vi "7Zip.vi"(6 "error in":errorcluster, 7 "Zip file Dir":path caption="Папка, в которую надо сложить архив", 8 "7za Dir":path caption="Папка, в которо лежит 7za.exe архиватор", 9 "File":path caption="Полный путь до файла, который надо зажать") -> (0 "error out":errorcluster, 1 "return code":i32, 2 "standard error":string, 3 "standard output":string="\r\n", 4 "new path":path caption="Полный путь до перемещённого архива файла")   [LabVIEW 2010]
panel:
  # "Инструмент для сжатия файлов архиватором 7za.exe  \nhttp://www.7-zip.org/download.html (нужен для командной строки)\n------------------------------------------------------------------------------------------------\nУказанный файл сжимается архиватором, лежащим по указанному месту\nи переносится в указанную папку. \n\nЕсли файла нет - ошибка\nЕсли архиватора нет - ошибка\nЕсли папки, куда переместить файл нет - ошибка\n\nЕсли всё ок, то в конце нет ошибок и в \"new path: путь до перемещенного \nзажатого файла, который можно дальше отсылать.\n-----------------------------------------------------------------------------------------------\n\nверсия 1.0 \nБутымов Антон Ноябрь 2010"
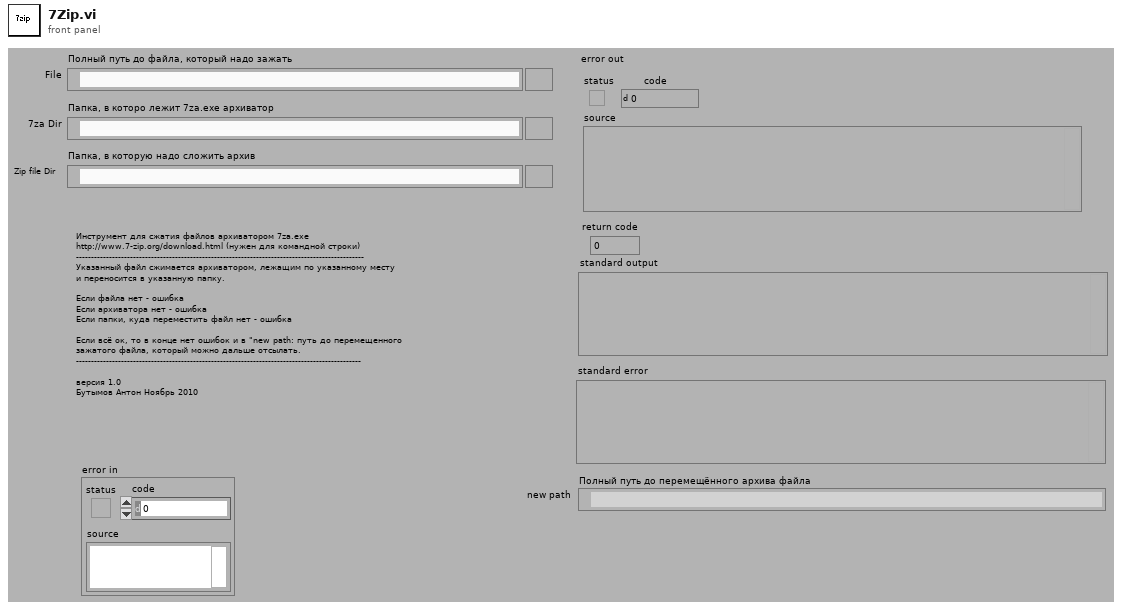
[diagram p1: front panel]
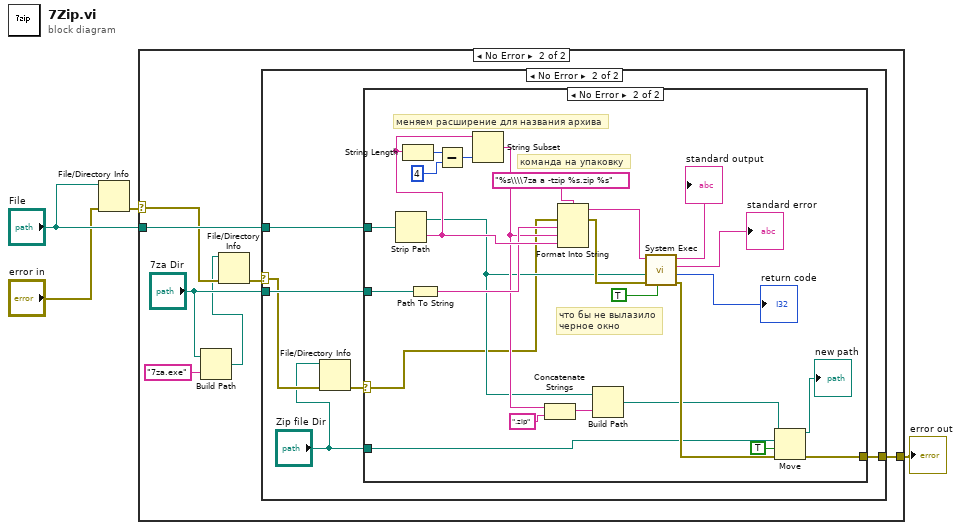
[diagram p0: block diagram]
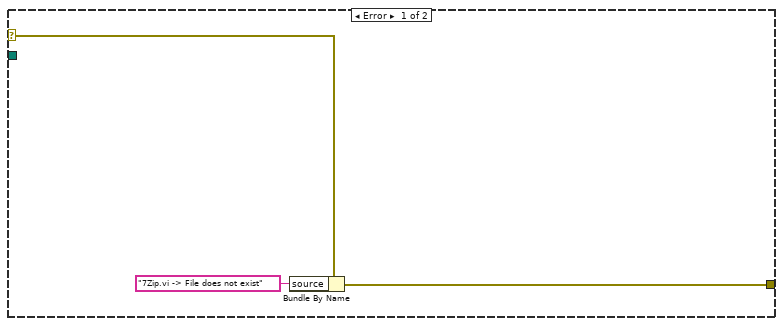
[diagram p2: hidden frame]
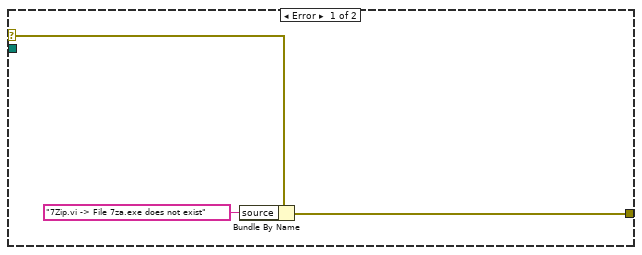
[diagram p3: hidden frame]
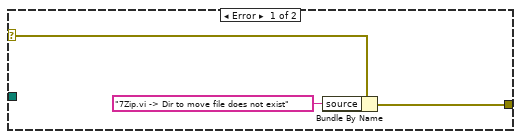
[diagram p4: hidden frame]
diagram:
  n1 = File/Directory Info(path="File", error in="error in") -> (error out=w2:errorcluster)  [unwired: 6 out]
  n2 = case shown="No Error" w2 {
    selector: w2 -> [w6 w12]
    tunnel: [w5 w14] -> w4
    tunnel: "File" -> [_ w13]
    frame Error {
      n3 = Bundle By Name(cluster=w6, "source"="7Zip.vi -> File does not exist") -> (w5:errorcluster)
    }
    frame No Error {
      n4 = Build Path(base path="7za Dir", name or relative path="7za.exe") -> (appended path=w8:path)
      n5 = File/Directory Info(path=w8, error in=w12) -> (error out=w11:errorcluster)  [unwired: 6 out]
      n6 = case shown="No Error" w11 {
        selector: w11 -> [w16 w20]
        tunnel: [w15 w23] -> w14
        tunnel: w13 -> [_ w22]
        tunnel: "7za Dir" -> [_ w21]
        frame Error {
          n7 = Bundle By Name(cluster=w16, "source"="7Zip.vi -> File 7za.exe does not exist") -> (w15:errorcluster)
        }
        frame No Error {
          n8 = File/Directory Info(path="Zip file Dir", error in=w20) -> (error out=w18:errorcluster)  [unwired: 6 out]
          n9 = case shown="No Error" w18 {
            selector: w18 -> [w26 w28]
            tunnel: [w25 w38] -> w23
            tunnel: w22 -> [_ w31]
            tunnel: w21 -> [_ w30]
            tunnel: "Zip file Dir" -> [_ w29]
            frame Error {
              n10 = Bundle By Name(cluster=w26, "source"="7Zip.vi -> Dir to move file does not exist") -> (w25:errorcluster)
            }
            frame No Error {
              # "что бы не вылазило\nчерное окно"
              # "команда на упаковку"
              # "меняем расширение для названия архива"
              n11 = Strip Path(path=w31) -> (stripped path=w34:path, name=w41:string)
              n12 = String Length(string=w41) -> (length=w44:i32)
              n13 = Path To String(path=w30) -> (string=w40:string)
              n14 = Subtract(x=w44, y=4) -> (x-y=w42:i32)
              n15 = String Subset(string=w41, length (rest)=w42) -> (substring=w37:string)  [unwired: 1 in]
              n16 = Concatenate Strings(w37, ".zip" ("string")) -> (w35:string)
              n17 = Format Into String(format string="%s\\\\7za a -tzip %s.zip %s" ("command line"), error in=w28, w40, w37, w41) -> (resulting string=w45:string, error out=w46:errorcluster)  [unwired: 1 in]
              n18 = Build Path(base path=w34, name or relative path=w35) -> (appended path=w33:path)
              n19 = call <vilib>:"System Exec.vi"("run minimized? (F)"=TRUE, "error in (no error)"=w46, "working directory"=w34, "command line"=w45) -> ("error out"=w39:errorcluster, "return code"=→"return code":i32, "standard error"=→"standard error":string, "standard output"=→"standard output":string)  [unwired: 4 in]
              n20 = Move(source path=w33, error in=w39, 9:TRUE ("overwrite (F)"), 10:w29) -> (error out=w38:errorcluster, 3:→"new path":path)  [unwired: 1 in, 1 out]
            }
          }
        }
      }
    }
  }
  "error out" <- w4
